vi "oa_Get DSA 446x Oversample Rate and Filter Delay.vi"(9 "EAR enabled? (F)":bool, 11 "vibration signal sample rate":dbl) -> (1 "start":dbl, 3 "oversample rate":dbl format="%#_6f")   [LabVIEW 2017, in "SoundVib_TachProcess.lvlib"]
uses:
  <vilib>/addons/Sound and Vibration/Order Analysis/Tach Process/SoundVib_TachProcess.lvlib
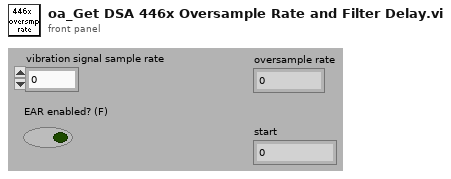
[diagram p1: front panel]
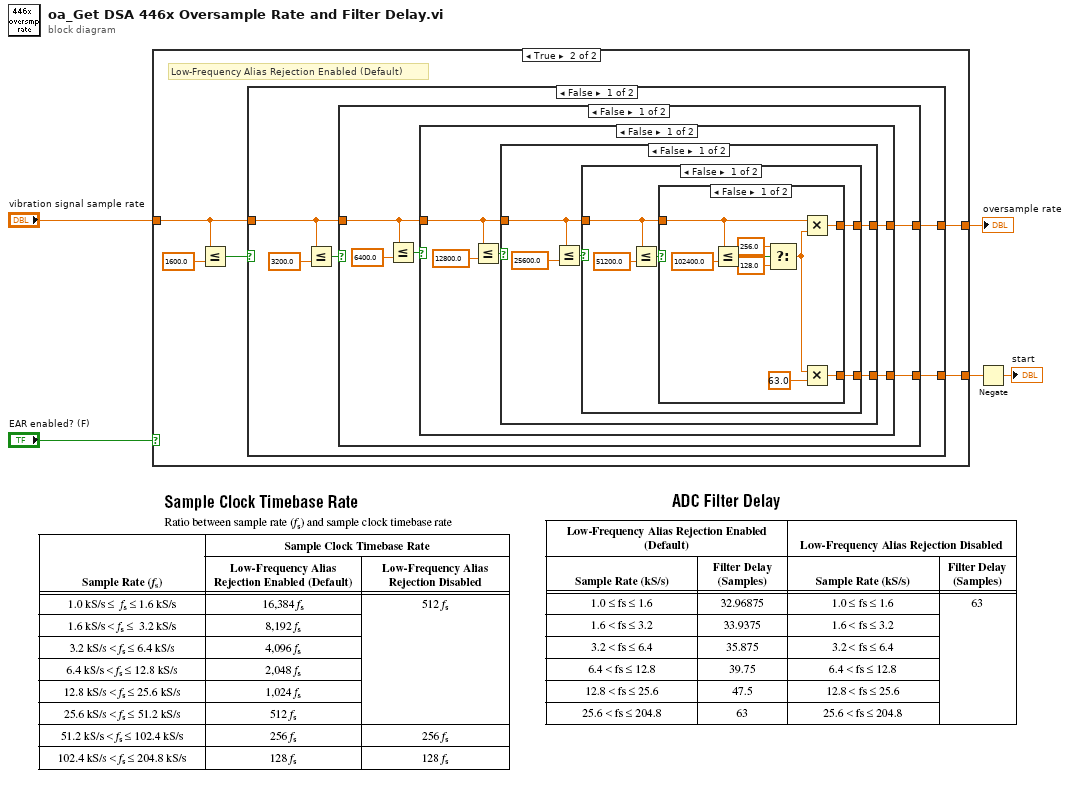
[diagram p0: block diagram]
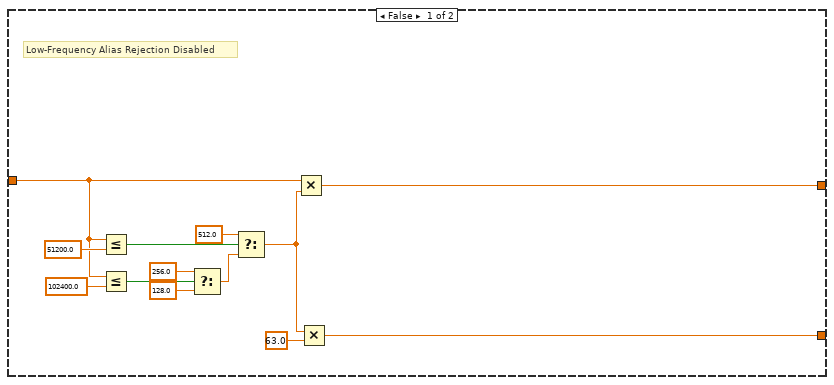
[diagram p2: hidden frame]
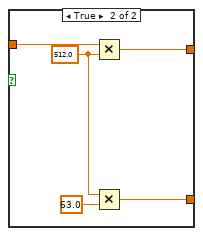
[diagram p3: hidden frame]
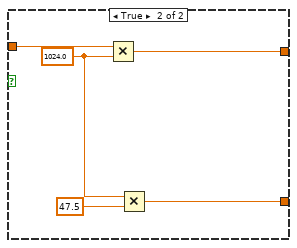
[diagram p4: hidden frame]
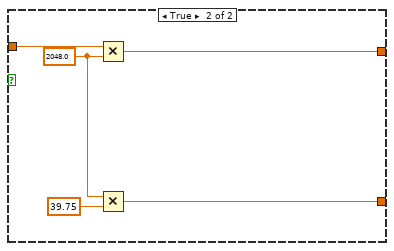
[diagram p5: hidden frame]
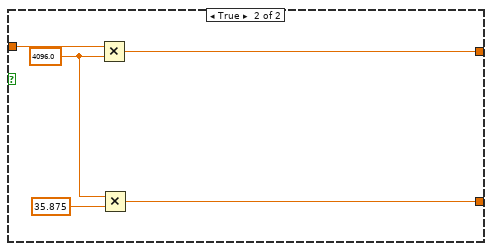
[diagram p6: hidden frame]
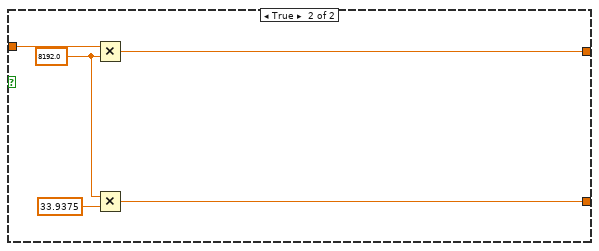
[diagram p7: hidden frame]
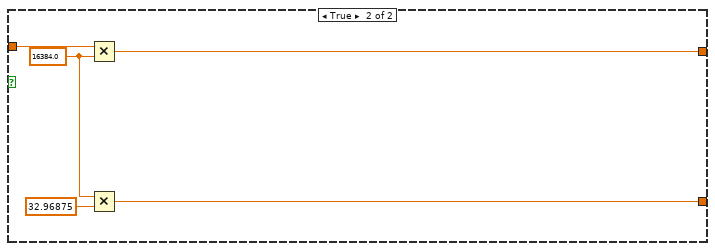
[diagram p8: hidden frame]
diagram:
  n1 = case shown="True" "EAR enabled? (F)" {
    tunnel: "vibration signal sample rate" -> [w12 w21]
    tunnel: [w14 w19] -> w1
    tunnel: [w13 w20] -> w2
    frame False {
      # "Low-Frequency Alias Rejection Disabled"
      n2 = Less Or Equal?(x=w12, y=51200.0) -> (x <= y?=w17:bool)
      n3 = Less Or Equal?(x=w12, y=102400.0) -> (x <= y?=w10:bool)
      n4 = Select(t=256.0, s=w10, f=128.0) -> (s? t:f=w7:dbl)
      n5 = Select(t=512.0, s=w17, f=w7) -> (s? t:f=w6:dbl)
      n6 = Multiply(x=w12, y=w6) -> (x*y=w13:dbl)
      n7 = Multiply(x=w6, y=63.0) -> (x*y=w14:dbl)
    }
    frame True {
      # "Low-Frequency Alias Rejection Enabled (Default)"
      n8 = Less Or Equal?(x=w21, y=1600.0) -> (x <= y?=w22:bool)
      n9 = case shown="False" w22 {
        tunnel: w21 -> [w26 w87]
        tunnel: [w25 w86] -> w20
        tunnel: [w24 w83] -> w19
        frame False {
          n10 = Less Or Equal?(x=w26, y=3200.0) -> (x <= y?=w27:bool)
          n11 = case shown="False" w27 {
            tunnel: w26 -> [w31 w82]
            tunnel: [w30 w81] -> w25
            tunnel: [w29 w78] -> w24
            frame False {
              n12 = Less Or Equal?(x=w31, y=6400.0) -> (x <= y?=w32:bool)
              n13 = case shown="False" w32 {
                tunnel: w31 -> [w36 w77]
                tunnel: [w35 w75] -> w30
                tunnel: [w34 w73] -> w29
                frame False {
                  n14 = Less Or Equal?(x=w36, y=12800.0) -> (x <= y?=w37:bool)
                  n15 = case shown="False" w37 {
                    tunnel: w36 -> [w41 w72]
                    tunnel: [w40 w71] -> w35
                    tunnel: [w39 w68] -> w34
                    frame False {
                      n16 = Less Or Equal?(x=w41, y=25600.0) -> (x <= y?=w42:bool)
                      n17 = case shown="False" w42 {
                        tunnel: w41 -> [w46 w67]
                        tunnel: [w45 w66] -> w40
                        tunnel: [w44 w63] -> w39
                        frame False {
                          n18 = Less Or Equal?(x=w46, y=51200.0) -> (x <= y?=w47:bool)
                          n19 = case shown="False" w47 {
                            tunnel: w46 -> [w53 w62]
                            tunnel: [w52 w61] -> w45
                            tunnel: [w51 w58] -> w44
                            frame False {
                              n20 = Less Or Equal?(x=w53, y=102400.0) -> (x <= y?=w56:bool)
                              n21 = Select(t=256.0, s=w56, f=128.0) -> (s? t:f=w50:dbl)
                              n22 = Multiply(x=w53, y=w50) -> (x*y=w52:dbl)
                              n23 = Multiply(x=w50, y=63.0) -> (x*y=w51:dbl)
                            }
                            frame True {
                              w60 = 512.0 ("y")
                              n24 = Multiply(x=w62, y=w60) -> (x*y=w61:dbl)
                              n25 = Multiply(x=w60, y=63.0) -> (x*y=w58:dbl)
                            }
                          }
                        }
                        frame True {
                          w65 = 1024.0 ("y")
                          n26 = Multiply(x=w67, y=w65) -> (x*y=w66:dbl)
                          n27 = Multiply(x=w65, y=47.5) -> (x*y=w63:dbl)
                        }
                      }
                    }
                    frame True {
                      w70 = 2048.0 ("y")
                      n28 = Multiply(x=w72, y=w70) -> (x*y=w71:dbl)
                      n29 = Multiply(x=w70, y=39.75) -> (x*y=w68:dbl)
                    }
                  }
                }
                frame True {
                  w74 = 4096.0 ("y")
                  n30 = Multiply(x=w77, y=w74) -> (x*y=w75:dbl)
                  n31 = Multiply(x=w74, y=35.875) -> (x*y=w73:dbl)
                }
              }
            }
            frame True {
              w80 = 8192.0 ("y")
              n32 = Multiply(x=w82, y=w80) -> (x*y=w81:dbl)
              n33 = Multiply(x=w80, y=33.9375) -> (x*y=w78:dbl)
            }
          }
        }
        frame True {
          w85 = 16384.0 ("y")
          n34 = Multiply(x=w87, y=w85) -> (x*y=w86:dbl)
          n35 = Multiply(x=w85, y=32.96875) -> (x*y=w83:dbl)
        }
      }
    }
  }
  "oversample rate" <- w2
  n36 = Negate(x=w1) -> (-x=→"start":dbl)
